vi "Write Data Word.vi"(4 "Data Word to Write":u16, 6 "Word Position":u8, 8 "Error In":errorcluster, 9 "Buffer Type":T1(ring)=enum."BC Message Buffer", 10 "Buffer Header and Buffer ID":u16=1, 11 "Module Handle":u32) -> (0 "Error Out":errorcluster, 3 "Module Handle out":u32)   [LabVIEW 2020, in "AIM MIL-STD-1553 Hardware API.lvlib"]
uses:
  AIM MIL-STD-1553 Hardware API.lvlib
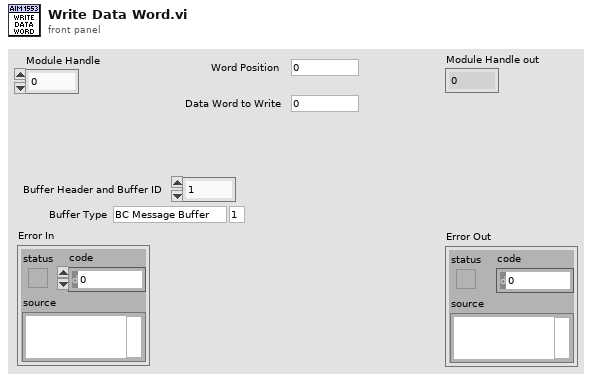
[diagram p1: front panel]
types:
  T1 = enum16{"unknown", "BC Message Buffer", "RT Message Buffer"}
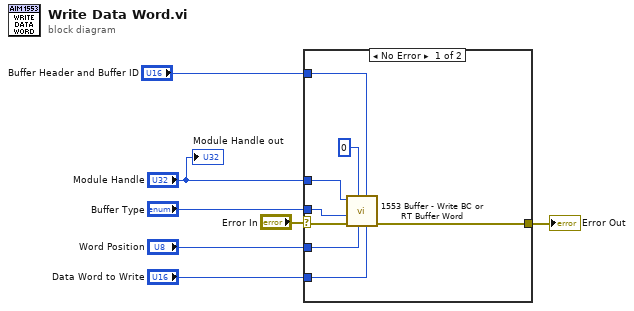
[diagram p0: block diagram]
diagram:
  n1 = case shown="No Error" "Error In" {
    selector: "Error In" -> [w15 w16]
    tunnel: [w11 w16] -> w7
    tunnel: "Module Handle" -> [w14 _]
    tunnel: "Buffer Type" -> [w13 _]
    tunnel: "Buffer Header and Buffer ID" -> [w9 _]
    tunnel: "Word Position" -> [w12 _]
    tunnel: "Data Word to Write" -> [w10 _]
    frame No Error {
      n2 = call <instrlib>:"1553 Buffer - Write BC or RT Buffer Word.vi"("Data Word to Write (0)"=w10, "Buffer ID (1)"=w9, "Word Position (0)"=w12, "Buffer Header ID (1)"=u16 0, "Error In (none)"=w15, "Buffer Type (BC)"=w13, "Module Handle"=w14) -> ("Error Out"=w11:errorcluster)  [unwired: 4 in]
    }
    frame Error {
    }
  }
  "Error Out" <- w7
  "Module Handle out" <- "Module Handle"
